vi "TCP IP Write.vi"(8 "error in (no error)":errorcluster, 10 "Data in":i32[](array[numeric]), 11 "TCP Network Connection in":refnum<k5>) -> (0 "error out":errorcluster, 3 "Write Data":dbl)   [LabVIEW 2017]
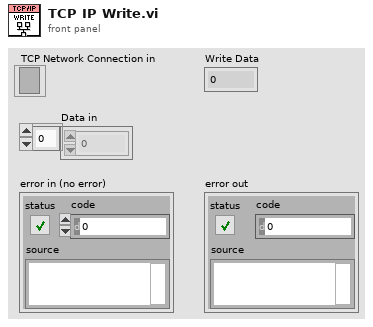
[diagram p1: front panel]
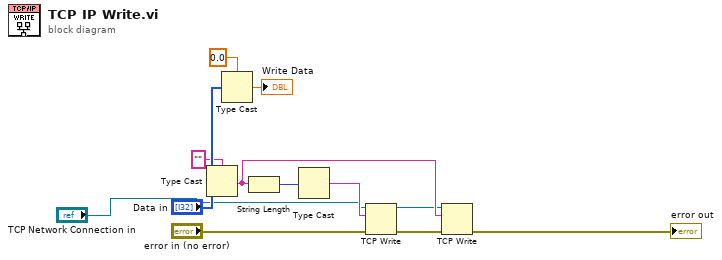
[diagram p0: block diagram]
diagram:
  n1 = Type Cast(type="", x="Data in") -> (*(type *) &x=w6:string)
  n2 = Type Cast(type=0.0, x="Data in") -> (*(type *) &x=→"Write Data":dbl)
  n3 = String Length(string=w6) -> (length=w7:i32)
  n4 = Type Cast(x=w7) -> (*(type *) &x=w8:string)  [unwired: 1 in]
  n5 = TCP Write(connection ID="TCP Network Connection in", data in=w8, error in (no error)="error in (no error)") -> (connection ID out=w5:refnum<k5>, error out=w4:errorcluster)  [unwired: 1 in, 1 out]
  n6 = TCP Write(connection ID=w5, data in=w6, error in (no error)=w4) -> (error out=→"error out":errorcluster)  [unwired: 1 in, 2 out]
